vi "WXA100 data insert.vi"(8 "error in (no error)":errorcluster, 11 "data":T1) -> (0 "error out":errorcluster)   [LabVIEW 2016, in "AIRMAR WeatherCaster.lvlib"]
uses:
  AIRMAR WeatherCaster.lvlib
panel:
  in  "data in":T2
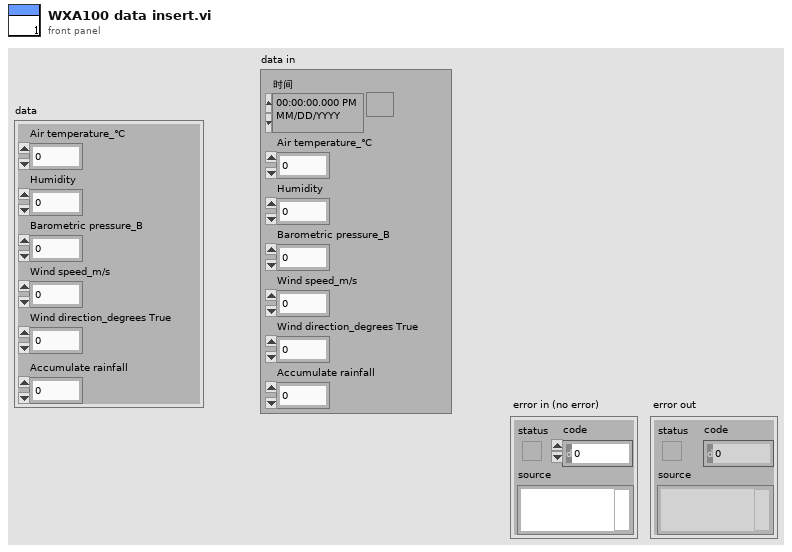
[diagram p1: front panel]
types:
  T1 = cluster{"Air temperature_℃":sgl, "Humidity":sgl, "Barometric pressure_B":sgl, "Wind speed_m/s":sgl, "Wind direction_degrees True":sgl, "Accumulate rainfall":sgl}
  T2 = cluster{"时间":timestamp, "Air temperature_℃":sgl, "Humidity":sgl, "Barometric pressure_B":sgl, "Wind speed_m/s":sgl, "Wind direction_degrees True":sgl, "Accumulate rainfall":sgl}
  T3 = typedef "数据库类型.ctl" = enum16{"Access", "SQLite"}
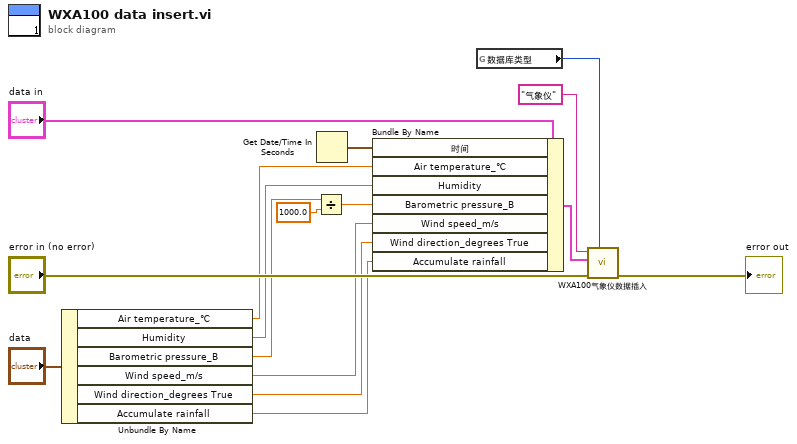
[diagram p0: block diagram]
diagram:
  n1 = Unbundle By Name("data") -> ("Air temperature_℃"=w9:sgl, "Humidity"=w8:sgl, "Barometric pressure_B"=w4:sgl, "Wind speed_m/s"=w7:sgl, "Wind direction_degrees True"=w6:sgl, "Accumulate rainfall"=w1:sgl)
  n2 = Divide(x=w4, y=sgl 1000.0) -> (x/y=w2:sgl)
  n3 = Get Date/Time In Seconds() -> (seconds since 1Jan1904=w11:timestamp)
  n4 = Bundle By Name(cluster="data in", "时间"=w11, "Air temperature_℃"=w9, "Humidity"=w8, "Barometric pressure_B"=w2, "Wind speed_m/s"=w7, "Wind direction_degrees True"=w6, "Accumulate rainfall"=w1) -> (w5:T2)
  n5 = global read "气象全局变量.vi" "数据库类型"() -> (w13:T3)
  n6 = call "WXA100气象仪数据插入.vi"("Tabe Name"="气象仪" ("table"), "data"=w5, "错误输入（无错误）"="error in (no error)", "数据库类型"=w13) -> ("错误输出"=→"error out":errorcluster)  [unwired: 6 in]
